vi "RouteGetOwner.vi"(10 "Route":string) -> (2 "Owner":string)   [LabVIEW 2012]
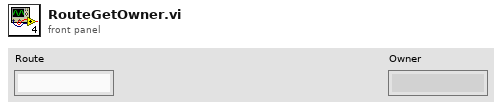
[diagram p1: front panel]
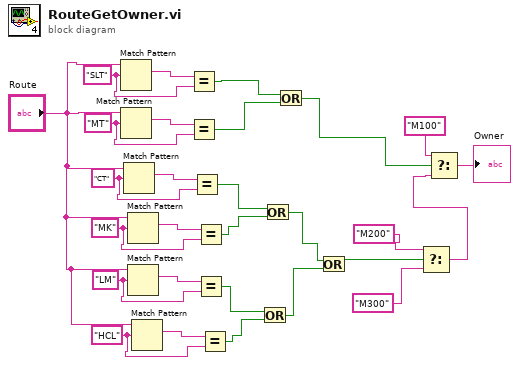
[diagram p0: block diagram]
diagram:
  w6 = "SLT" ("regular expression")
  w20 = "HCL" ("regular expression")
  w21 = "LM" ("regular expression")
  w24 = "MK" ("regular expression")
  w25 = "CT" ("regular expression")
  w27 = "MT" ("regular expression")
  n1 = Match Pattern(string="Route", regular expression=w6) -> (match substring=w5:string)  [unwired: 1 in, 3 out]
  n2 = Match Pattern(string="Route", regular expression=w27) -> (match substring=w28:string)  [unwired: 1 in, 3 out]
  n3 = Match Pattern(string="Route", regular expression=w25) -> (match substring=w26:string)  [unwired: 1 in, 3 out]
  n4 = Match Pattern(string="Route", regular expression=w24) -> (match substring=w23:string)  [unwired: 1 in, 3 out]
  n5 = Match Pattern(string="Route", regular expression=w21) -> (match substring=w22:string)  [unwired: 1 in, 3 out]
  n6 = Match Pattern(string="Route", regular expression=w20) -> (match substring=w19:string)  [unwired: 1 in, 3 out]
  n7 = Equal?(x=w5, y=w6) -> (x = y?=w3:bool)
  n8 = Equal?(x=w28, y=w27) -> (x = y?=w2:bool)
  n9 = Equal?(x=w26, y=w25) -> (x = y?=w18:bool)
  n10 = Equal?(x=w23, y=w24) -> (x = y?=w17:bool)
  n11 = Equal?(x=w22, y=w21) -> (x = y?=w16:bool)
  n12 = Equal?(x=w19, y=w20) -> (x = y?=w15:bool)
  n13 = Or(x=w16, y=w15) -> (x .or. y?=w13:bool)
  n14 = Or(x=w18, y=w17) -> (x .or. y?=w14:bool)
  n15 = Or(x=w3, y=w2) -> (x .or. y?=w1:bool)
  n16 = Or(x=w14, y=w13) -> (x .or. y?=w11:bool)
  n17 = Select(t="M200", s=w11, f="M300") -> (s? t:f=w8:string)
  n18 = Select(t="M100", s=w1, f=w8) -> (s? t:f=→"Owner":string)
